vi "Image Processing.vi"() -> ()   [LabVIEW 2016]
uses:
  <vilib>/rvi/Emulation/niFpgaGetClockAttributes.vi
  <vilib>/rvi/Emulation/niFpgaSctlEmulationGetInTimedLoop.vi
  <vilib>/rvi/Emulation/niFpgaEmulationReportErrorSimple.vi
  <vilib>/rvi/Emulation/niFpgaProcessEmulError.vi
  <vilib>/rvi/eio/common/nirviEmuTemplateMethod_errors.vi
  <vilib>/rvi/interface/RandomDataEmulation/niFpgaRandomDataHandleErrors.vi
  <vilib>/rvi/DataTransferAndStorage/Container/Common/niFpgaContainerGetUniqueNameForEmu.vi
  <vilib>/rvi/DataTransferAndStorage/Container/Common/niFpgaContainerSetEmuInfo.vi
  <vilib>/rvi/eio/common/nirviEmuReportErrorAndStop.vi
  <vilib>/rvi/DataTransferAndStorage/Container/Common/niFpgaContainerExecOnDevCompGetState.vi
  <vilib>/rvi/Emulation/niFpgaEmulationIsFPGAContextNoSignature.vi
  <vilib>/rvi/errors/niFpgaSetErrorForExecOnDevCompSimple.vi
  <vilib>/rvi/FIFO/Fifo_Resource/nirvififoEmulationSetSize.vi
  <vilib>/rvi/FIFO/Fifo_Resource/nirviFifoEmulationQueueMgr.vi
  <instcachedir>/0/nirviFifoEmulationQueueMgr_E5CAEC123FF24DC58D834DCA3CDAA9B5.lvgen/nirviFifoEmulationQueueMgr_E5CAEC123FF24DC58D834DCA3CDAA9B5_002.vi
  <vilib>/rvi/FIFO/Fifo_Resource/nirvififoEmulationDetermineInputValidOut.vi
  <vilib>/rvi/FIFO/Fifo_Resource/nirvififoEmulationCreateLock.vi
  <vilib>/rvi/FIFO/Fifo_Resource/nirvififoEmulationObtainLock.vi
  <vilib>/rvi/FIFO/Fifo_Resource/nirvififoEmulationReleaseLock.vi
  <vilib>/rvi/occurrence/nirviWaitOnOccurrenceBase.vi
  <vilib>/rvi/errors/nirviReportUnexpectedCaseInternalError.vi
  <vilib>/rvi/errors/nirviReportUnexpectedCaseInternalError (U32).vi
  <vilib>/Utility/error.llb/Clear Errors.vi
  <vilib>/rvi/Emulation/niFpgaCriticalErrorInLSC.vi
  <vilib>/eio/EIONode/EIONode.xnode
  <vilib>/rvi/DataTransferAndStorage/Container/XNode/niFpgaContainer.xnode
  <vilib>/rvi/interface/RandomDataEmulation/nirviRandomDataFpgaReadWriteTemplate.vi
  <vilib>/rvi/LocalResourceManager/LocalResourceManager.xnode
  <vilib>/rvi/FIFO/Fifo_Resource/niFpgaFifoEmulationRefIn.vi
panel:
  out "dec deHeight":u16
  out "dec deWidth":u16
  out "dec Height":u16
  out "dec Width":u16
  out "Width":u16=320
  out "Height":u16=240
  out "deHeight":u16=240
  out "deWidth":u16=320
  out "Count":u32
  out "OutputType":u8
  out "CanSendImage":bool=TRUE
  out "Mode LED Status":bool=TRUE
  out "Radio LED Status":bool=TRUE
  out "outputExtreme2":bool=TRUE
  out "outputExtreme1":bool=TRUE
  out "outputDOG2":bool=TRUE
  out "outputDOG1":bool=TRUE
  out "Ready For Output":bool=TRUE
  out "StartOfImage":bool=TRUE
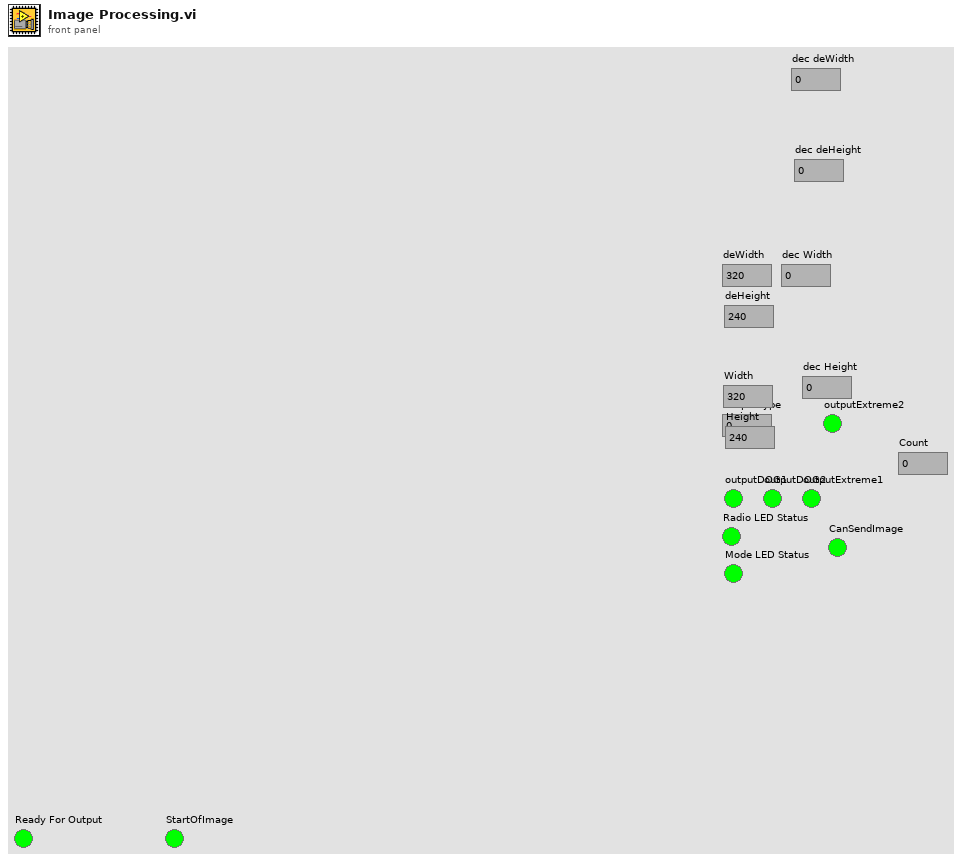
[diagram p1: front panel]
types:
  T1 = cluster{"curCol":u16, "curRow":u16, "Width":u16, "Height":u16, "Data Out":u8, bool}
  T2 = cluster{"curCol":u16, "curRow":u16, "Width":u16, "Height":u16, "GaussianFilterData out":u8, "DV out":bool}
  T3 = cluster{"t":i16, "t":i16, "deWidth":u16, "deHeight":u16, "GaussianFilterData out":u8, "DV out":bool}
  T4 = cluster{"t":i16, "t":i16, "deWidth":u16, "deHeight":u16, "Data Out":u8, "DV out":bool}
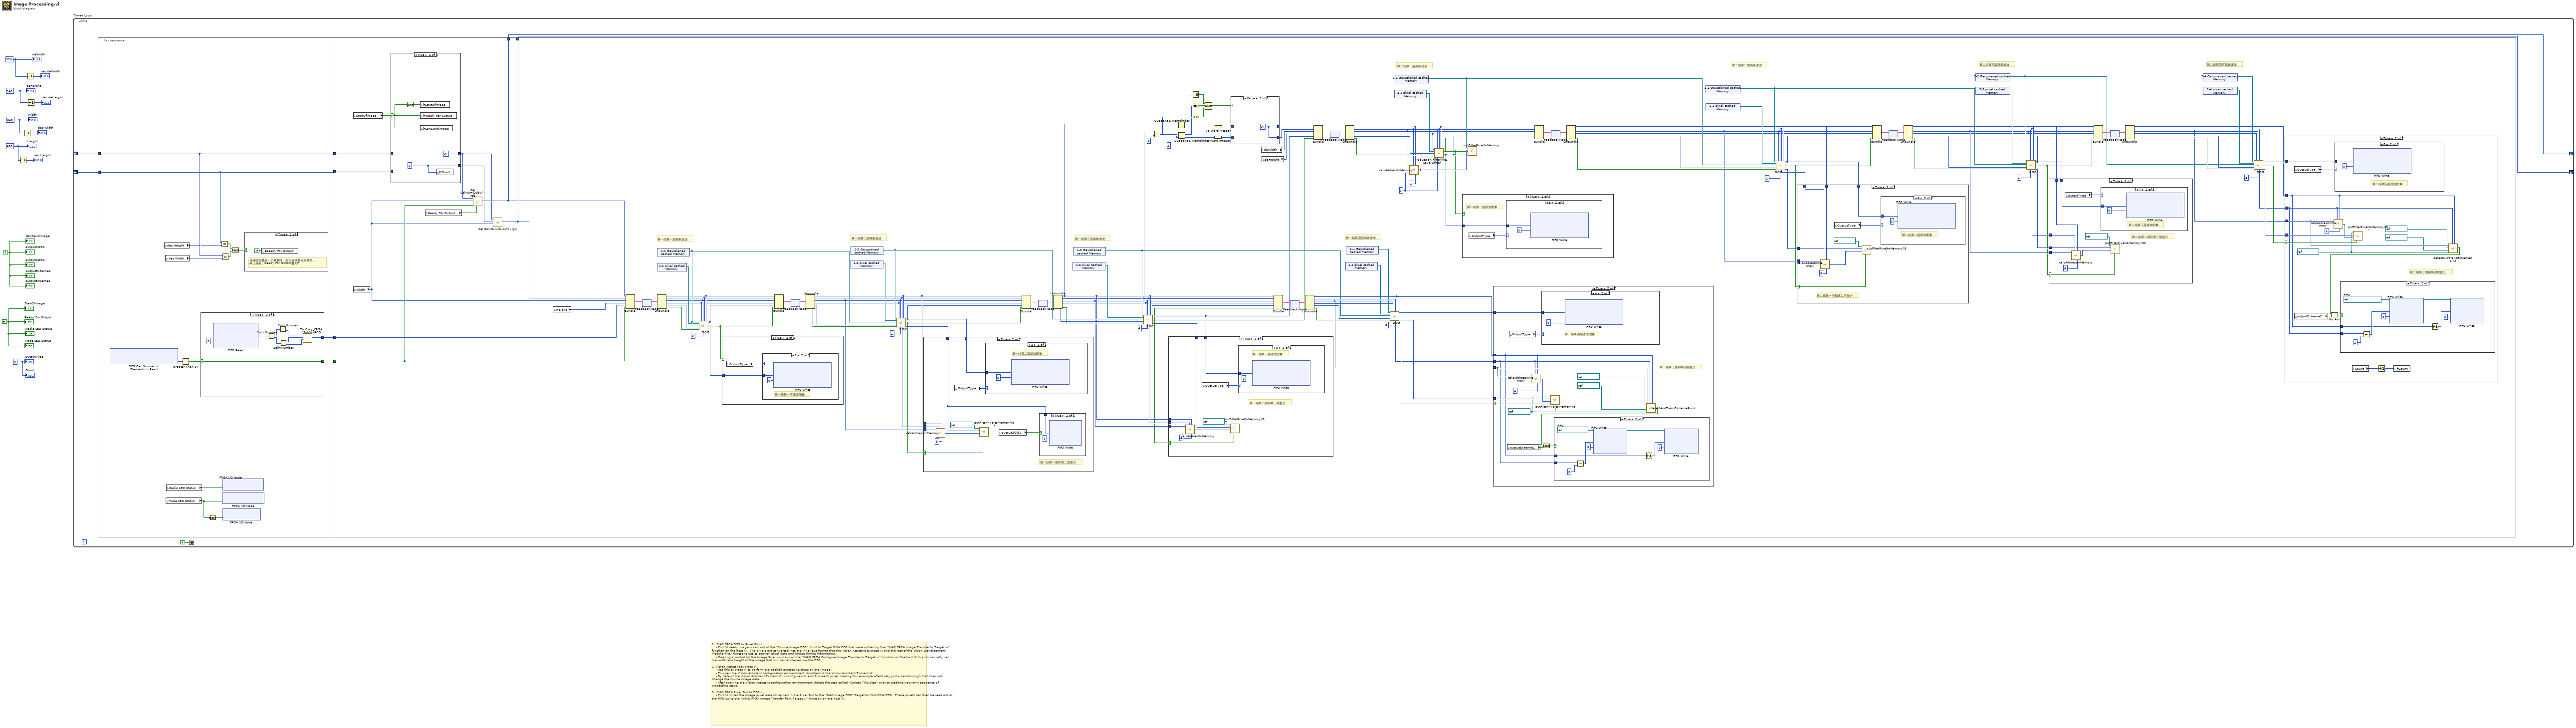
[diagram p0: block diagram]
diagram:
  w5 = i16 480
  w8 = i16 640
  w1 = i16 240
  w3 = i16 320
  w9 = FALSE
  w10 = i16 0
  w11 = TRUE ("Ready For Output")
  # "1. IMAQ FPGA FIFO to Pixel Bus.vi\n    - This VI reads image pixels out of the \"Source Image FIFO\"  Host to Target DMA FIFO that were written by the \"IMAQ FPGA Image Transfer to Target.vi\" function on the host VI.  The pixels are converted into the Pixel Bus format that the Vision Assistant Express VI and the rest of the Vision Development Module FPGA functions use to convey pixel data and image timing information.\n    - Creating a control for the Image Size input allows the \"IMAQ FPGA Configure Image Transfer to Target.vi\" function on the host VI to automatically set the width and height of the image that will be transferred via the FIFO.\n\n2. Vision Assistant Express VI\n    - Use this Express VI to perform the desired processing steps on the image.\n    - To open the Vision Assistant configuration environment, double-click the Vision Assistant Express VI.\n    - By default the Vision Assistant Express VI is configured to add 0 to each pixel, making this example effectively just a pass-through that does not change the source image data.\n    - After opening the Vision Assistant configuration environment, delete the step called \"Delete This Step\" prior to creating your own sequence of processing steps.\n\n3. IMAQ FPGA Pixel Bus to FIFO.vi\n    - This VI writes the image pixel data contained in the Pixel Bus to the \"Dest Image FIFO\" Target to Host DMA FIFO.  These pixels can then be read out of the FIFO using the \"IMAQ FPGA Image Transfer from Target.vi\" function on the host VI."
  n1 = Decrement(x=w5) -> (x-1=→"dec Height":i16)
  n2 = Decrement(x=w8) -> (x-1=→"dec Width":i16)
  n3 = Decrement(x=w3) -> (x-1=→"dec deWidth":i16)
  n4 = Decrement(x=w1) -> (x-1=→"dec deHeight":i16)
  n5 = while "Timed Loop" {
    shift-right: [w12] -> _
    shift-left: _ -> [w14]
    shift-right: [w13] -> _
    shift-left: _ -> [w16]
    stop <- FALSE stop-if-true
    n6 = flat-sequence {
      tunnel: [w29] -> w19
      tunnel: [w28] -> w18
      tunnel: [w23] -> w17
      tunnel: w16 -> [w23]
      tunnel: [w24] -> w15
      tunnel: w14 -> [w24]
      tunnel: w19 -> [w115]
      tunnel: w18 -> [w114]
      tunnel: w17 -> [w49]
      tunnel: w15 -> [w48]
      tunnel: [w55] -> w12
      tunnel: [w54] -> w13
      frame #0 {
        n7 = xnode ("FIFO Get Number of Elements to Read")() -> ("Number of Elements to Read"=w31:u32)  [unwired: 1 in, 1 out]
        n8 = local read "dec Height"() -> (w22:u16)
        n9 = local read "dec Width"() -> (w21:u16)
        n10 = local read "Mode LED Status"() -> (w34:bool)
        n11 = local read "Radio LED Status"() -> (w32:bool)
        n12 = Greater Than 0?(x=w31) -> (x > 0?=w30:bool)
        n13 = case shown="True" w30 {
          selector: w30 -> [w36 w37]
          tunnel: [_ w38] -> w29
          tunnel: [w36 w37] -> w28
          frame False {
          }
          frame True {
            n14 = xnode ("FIFO Read")("Timeout"=0) -> ("Element"=w45:u32)  [unwired: 1 in, 2 out]
            n15 = Split Number(x=w45) -> (hi(x)=w43:u16, lo(x)=w44:u16)
            n16 = Split Number(x=w43) -> (lo(x)=w42:u8)  [unwired: 1 out]
            n17 = Split Number(x=w44) -> (hi(x)=w41:u8, lo(x)=w40:u8)
            n18 = call "To Gray_FPGA (SubVI)-RGB.vi"("B"=w40, "G"=w41, "R"=w42) -> ("Data Out"=w38:u8)  [unwired: 8 in]
          }
        }
        n19 = Not(x=w34) -> (.not. x?=w33:bool)
        n20 = Equal?(x=w24, y=w22) -> (x = y?=w25:bool)
        n21 = Equal?(x=w23, y=w21) -> (x = y?=w26:bool)
        n22 = xnode "FPGA I/O Node"("Radio LED Green"=w32) -> ()  [unwired: 1 in, 1 out]
        n23 = xnode "FPGA I/O Node"("Mode LED Green"=w34) -> ()  [unwired: 1 in, 1 out]
        n24 = xnode "FPGA I/O Node"("Mode LED Red"=w33) -> ()  [unwired: 1 in, 1 out]
        n25 = And(x=w25, y=w26) -> (x .and. y?=w27:bool)
        n26 = case shown="True" w27 {
          frame False {
          }
          frame True {
            # "当接收完最后一个像素时，由于后续差分未做完，\n停止接收，Ready For Output置为F"
            n27 = local write "Ready For Output"(FALSE ("Ready For Output")) -> ()
          }
        }
      }
      frame #1 {
        w138 = u32 2 ("y")
        w146 = u8 0 ("delayRowCount")
        # "第一组第一层高斯滤波"
        # "第一组第二层高斯滤波"
        # "第一组第三层高斯滤波"
        # "第二组第一层高斯滤波"
        # "第一组第四层高斯滤波"
        # "第二组第二层高斯滤波"
        # "第二组第三层高斯滤波"
        # "第二组第四层高斯滤波"
        n28 = local read "StartOfImage"() -> (w50:bool)
        n29 = local read "Width"() -> (w47:u16)
        n30 = case shown="True" w50 {
          selector: w50 -> [_ w196]
          tunnel: w49 -> [w194 _]
          tunnel: w48 -> [w193 _]
          tunnel: [w194 i16 -1] -> w52
          tunnel: [w193 w195] -> w51
          frame False {
          }
          frame True {
            w195 = i16 0
            n31 = Not(x=w196) -> (.not. x?=w197:bool)
            n32 = local write "StartOfImage"(w197) -> ()
            n33 = local write "Ready For Output"(w196) -> ()
            n34 = local write "CanSendImage"(w196) -> ()
            n35 = local write "Count"(w195) -> ()
          }
        }
        n36 = local read "Ready For Output"() -> (w53:bool)
        n37 = call "Cal ColNum(SubVI) - rgb.vi"("Ready For Input"=w53, "DV"=w114, "Width"=w47, "preCol"=w52) -> ("curCol"=w54:u16)  [unwired: 7 in]
        n38 = call "Cal RowNum(SubVI) - rgb.vi"("Width"=w47, "preRow"=w51, "preCol"=w52) -> ("curRow"=w55:u16)  [unwired: 8 in]
        n39 = local read "Height"() -> (w46:u16)
        n40 = Bundle("curCol"=w54, "curRow"=w55, "Width"=w47, "Height"=w46, "Data Out"=w115, w114) -> (w119:T1)  [unwired: 1 in]
        n41 = feedback #1() -> (w118:T1)  [unwired: 1 in]
        n42 = feedback-in #1(w119) -> ()
        n43 = xnode "1-1 Gaussianed cached Memory"() -> ("Memory Out"=w126:refnum<k21>)
        n44 = xnode "1-1 pixel cached Memory"() -> ("Memory Out"=w121:refnum<k21>)
        n45 = Unbundle(w118) -> ("curCol"=w111:u16, "curRow"=w110:u16, "Width"=w109:u16, "Height"=w108:u16, "Data Out"=w117:u8, w116:bool)
        n46 = call "DOG.vi"("Gaussianed cached Memory"=w126, "pixel cached Memory"=w121, "preGaussianed cached Memory"=w126, "Data in"=w117, "DV in"=w116, "Height"=w108, "Width"=w109, "DelayRowCount"=i16 0, "Rows"=w110, "Cols"=w111) -> ("GaussianFilterData out"=w107:u8, "DV out"=w106:bool)  [unwired: 6 in, 2 out]
        n47 = case shown="True" w106 {
          tunnel: w107 -> [_ w200]
          frame False {
          }
          frame True {
            n48 = local read "OutputType"() -> (w199:u8)
            n49 = case shown="1" w199 {
              tunnel: w200 -> [_ w201]
              frame 0, Default {
              }
              frame 1 {
                # "第一组第一层滤波图像"
                n50 = xnode ("FIFO Write")("Element"=w201, "Timeout"=0) -> ()  [unwired: 1 in, 2 out]
              }
            }
          }
        }
        n51 = Bundle("curCol"=w111, "curRow"=w110, "Width"=w109, "Height"=w108, "GaussianFilterData out"=w107, "DV out"=w106) -> (w112:T2)  [unwired: 1 in]
        n52 = feedback #2() -> (w113:T2)  [unwired: 1 in]
        n53 = feedback-in #2(w112) -> ()
        n54 = Unbundle(w113) -> ("curCol"=w103:u16, "curRow"=w102:u16, "Width"=w101:u16, "Height"=w100:u16, "GaussianFilterData out"=w125:u8, "DV out"=w124:bool)
        n55 = xnode "1-2 Gaussianed cached Memory"() -> ("Memory Out"=w141:refnum<k21>)
        n56 = xnode "1-2 pixel cached Memory"() -> ("Memory Out"=w127:refnum<k21>)
        n57 = call "DOG.vi"("Gaussianed cached Memory"=w141, "pixel cached Memory"=w127, "preGaussianed cached Memory"=w126, "Data in"=w125, "DV in"=w124, "Height"=w100, "Width"=w101, "DelayRowCount"=i16 2, "Rows"=w102, "Cols"=w103) -> ("out Row"=w122:u16, "GaussianFilterData out"=w99:u8, "DV out"=w98:bool, "DOG Out"=w123:i8)  [unwired: 6 in]
        n58 = case shown="True" w98 {
          selector: w98 -> [_ w206]
          tunnel: w99 -> [_ w213]
          tunnel: w123 -> [_ w204]
          tunnel: w101 -> [_ w212]
          tunnel: w122 -> [_ w211]
          tunnel: w103 -> [_ w210]
          frame False {
          }
          frame True {
            # "第一组第一层和第二层差分"
            n59 = call "calcAddressInMemory.vi"("Width"=w212, "Rows"=w211, "Cols"=w210, "divider"=u8 8) -> ("addressInMemory"=w208:u16)  [unwired: 5 in]
            n60 = local read "OutputType"() -> (w205:u8)
            n61 = call "putFilterPixeltoMemory(I8).vi"("DV in"=w206, "addressInMemory"=w208, "Data In"=w204, "Memory in"=refnum<k21> "DOG1-1") -> ()  [unwired: 8 in]
            n62 = case shown="2" w205 {
              tunnel: w213 -> [_ w216]
              frame 0, Default {
              }
              frame 2 {
                # "第一组第二层滤波图像"
                n63 = xnode ("FIFO Write")("Element"=w216, "Timeout"=0) -> ()  [unwired: 1 in, 2 out]
              }
            }
            n64 = local read "outputDOG1"() -> (w203:bool)
            n65 = case shown="True" w203 {
              tunnel: w204 -> [_ w215]
              frame False {
              }
              frame True {
                n66 = xnode ("FIFO Write")("Element"=w215, "Timeout"=0) -> ()  [unwired: 1 in, 2 out]
              }
            }
          }
        }
        n67 = Bundle("curCol"=w103, "curRow"=w102, "Width"=w101, "Height"=w100, "GaussianFilterData out"=w99, "DV out"=w98) -> (w105:T2)  [unwired: 1 in]
        n68 = feedback #3() -> (w104:T2)  [unwired: 1 in]
        n69 = feedback-in #3(w105) -> ()
        n70 = Unbundle(w104) -> ("curCol"=w95:u16, "curRow"=w94:u16, "Width"=w93:u16, "Height"=w92:u16, "GaussianFilterData out"=w143:u8, "DV out"=w144:bool)
        n71 = xnode "1-3 pixel cached Memory"() -> ("Memory Out"=w142:refnum<k21>)
        n72 = xnode "1-3 Gaussianed cached Memory"() -> ("Memory Out"=w158:refnum<k21>)
        n73 = call "DOG.vi"("Gaussianed cached Memory"=w158, "pixel cached Memory"=w142, "preGaussianed cached Memory"=w141, "Data in"=w143, "DV in"=w144, "Height"=w92, "Width"=w93, "DelayRowCount"=i16 4, "Rows"=w94, "Cols"=w95) -> ("out Row"=w129:u16, "GaussianFilterData out"=w81:u8, "DV out"=w80:bool, "DOG Out"=w130:i8)  [unwired: 6 in]
        n74 = Subtract(x=w94, y=i16 6) -> (x-y=w133:u16)
        n75 = case shown="True" w80 {
          selector: w80 -> [_ w222]
          tunnel: w81 -> [_ w230]
          tunnel: w130 -> [_ w223]
          tunnel: w129 -> [_ w226]
          tunnel: w93 -> [_ w225]
          tunnel: w95 -> [_ w224]
          frame False {
          }
          frame True {
            # "第一组第二层和第三层差分"
            n76 = call "calcAddressInMemory.vi"("Width"=w225, "Rows"=w226, "Cols"=w224, "divider"=u8 6) -> ("addressInMemory"=w228:u16)  [unwired: 5 in]
            n77 = local read "OutputType"() -> (w221:u8)
            n78 = call "putFilterPixeltoMemory(I8).vi"("DV in"=w222, "addressInMemory"=w228, "Data In"=w223, "Memory in"=refnum<k21> "DOG1-2") -> ()  [unwired: 8 in]
            n79 = case shown="3" w221 {
              tunnel: w230 -> [_ w231]
              frame 0, Default {
              }
              frame 3 {
                # "第一组第三层滤波图像"
                n80 = xnode ("FIFO Write")("Element"=w231, "Timeout"=0) -> ()  [unwired: 1 in, 2 out]
              }
            }
          }
        }
        n81 = Quotient & Remainder(x=w95, y=w138) -> (x-y*floor(x/y)=w132:u32, floor(x/y)=w88:u32)
        n82 = Quotient & Remainder(x=w133, y=w138) -> (x-y*floor(x/y)=w131:u32, floor(x/y)=w86:u32)
        n83 = Equal To 0?(x=w132) -> (x = 0?=w137:bool)
        n84 = Equal To 0?(x=w131) -> (x = 0?=w136:bool)
        n85 = Greater Or Equal To 0?(x=w133) -> (x >= 0?=w135:bool)
        n86 = Compound Arithmetic op=AND(w137, w136, w135) -> (w134:bool)
        n87 = To Word Integer(number=w86) -> (16bit integer=w87:i16)
        n88 = To Word Integer(number=w88) -> (16bit integer=w89:i16)
        n89 = case shown="False" w134 {
          tunnel: [w218 w220] -> w85
          tunnel: w89 -> [_ w220]
          tunnel: [w218 w219] -> w84
          tunnel: w87 -> [_ w219]
          frame False {
            w218 = i16 -1 ("t")
          }
          frame True {
          }
        }
        n90 = local read "deWidth"() -> (w83:u16)
        n91 = local read "deHeight"() -> (w82:u16)
        n92 = Bundle("curCol"=w95, "curRow"=w94, "Width"=w93, "Height"=w92, "GaussianFilterData out"=w81, "DV out"=w80) -> (w96:T2)  [unwired: 1 in]
        n93 = feedback #4() -> (w97:T2)  [unwired: 1 in]
        n94 = feedback-in #4(w96) -> ()
        n95 = Unbundle(w97) -> ("curCol"=w148:u16, "curRow"=w162:u16, "Width"=w150:u16, "Height"=w161:u16, "GaussianFilterData out"=w164:u8, "DV out"=w163:bool)
        n96 = Bundle("t"=w85, "t"=w84, "deWidth"=w83, "deHeight"=w82, "GaussianFilterData out"=w81, "DV out"=w80) -> (w90:T3)  [unwired: 1 in]
        n97 = feedback #5() -> (w91:T3)  [unwired: 1 in]
        n98 = feedback-in #5(w90) -> ()
        n99 = Unbundle(w91) -> ("t"=w77:i16, "t"=w76:i16, "deWidth"=w75:u16, "deHeight"=w74:u16, "GaussianFilterData out"=w154:u8, "DV out"=w155:bool)
        n100 = xnode "1-4 pixel cached Memory"() -> ("Memory Out"=w159:refnum<k21>)
        n101 = xnode "1-4 Gaussianed cached Memory"() -> ("Memory Out"=w160:refnum<k21>)
        n102 = call "DOG.vi"("Gaussianed cached Memory"=w160, "pixel cached Memory"=w159, "preGaussianed cached Memory"=w158, "Data in"=w164, "DV in"=w163, "Height"=w161, "Width"=w150, "DelayRowCount"=i16 6, "Rows"=w162, "Cols"=w148) -> ("out Row"=w149:u16, "GaussianFilterData out"=w156:u8, "DV out"=w152:bool, "DOG Out"=w151:i8)  [unwired: 6 in]
        n103 = xnode "2-1 Gaussianed cached Memory"() -> ("Memory Out"=w169:refnum<k21>)
        n104 = xnode "2-1 pixel cached Memory"() -> ("Memory Out"=w153:refnum<k21>)
        n105 = call "calcAddressInMemory.vi"("Width"=w75, "Rows"=w76, "delayRowCount"=w146, "Cols"=w77, "divider"=u8 4) -> ("addressInMemory"=w147:u16)  [unwired: 4 in]
        n106 = call "Gaussian Filter(Pic1 LevelOther).vi"("Height"=w74, "Width"=w75, "Rows"=w76, "Cols"=w77, "Memory in"=w153, "Data in"=w154, "DV in"=w155, "Address In"=w147, "DelayRowCount"=w146) -> ("DV out"=w72:bool, "Data Out"=w73:u8)  [unwired: 4 in, 1 out]
        n107 = case shown="True" w72 {
          tunnel: w73 -> [_ w234]
          frame False {
          }
          frame True {
            # "第二组第一层滤波图像"
            n108 = local read "OutputType"() -> (w233:u8)
            n109 = case shown="5" w233 {
              tunnel: w234 -> [_ w235]
              frame 0, Default {
              }
              frame 5 {
                n110 = xnode ("FIFO Write")("Element"=w235, "Timeout"=0) -> ()  [unwired: 1 in, 2 out]
              }
            }
          }
        }
        n111 = call "putFilterPixeltoMemory.vi"("Data In"=w73, "DV in"=w72, "addressInMemory"=w147, "Memory in"=w169) -> ()
        n112 = case shown="True" w152 {
          selector: w152 -> [_ w247]
          tunnel: w156 -> [_ w251]
          tunnel: w151 -> [_ w248]
          tunnel: w150 -> [_ w246]
          tunnel: w149 -> [_ w240]
          tunnel: w148 -> [_ w241]
          frame False {
          }
          frame True {
            w243 = refnum<k21> "DOG1-3" ("Memory in")
            # "第一组第三层和第四层差分"
            n113 = local read "outputExtreme1"() -> (w238:bool)
            n114 = local read "OutputType"() -> (w242:u8)
            n115 = call "calcAddressInMemory.vi"("Width"=w246, "Rows"=w240, "Cols"=w241, "divider"=u8 4) -> ("addressInMemory"=w249:u16)  [unwired: 5 in]
            n116 = case shown="4" w242 {
              tunnel: w251 -> [_ w262]
              frame 0, Default {
              }
              frame 4 {
                # "第一组第四层滤波图像"
                n117 = xnode ("FIFO Write")("Element"=w262, "Timeout"=0) -> ()  [unwired: 1 in, 2 out]
              }
            }
            n118 = call "putFilterPixeltoMemory(I8).vi"("DV in"=w247, "addressInMemory"=w249, "Data In"=w248, "Memory in"=w243) -> ()  [unwired: 8 in]
            n119 = call "detectAndTransExtremePoint.vi"("Col"=w241, "Row"=w240, "Level3 Memory"=w243, "Level2 Memory"=refnum<k21> "DOG1-2" ("Memory In"), "Level1 Memory"=refnum<k21> "DOG1-1" ("Memory In"), "Width"=w246) -> ("isExtreme?"=w237:bool)  [unwired: 5 in]
            n120 = And(x=w237, y=w238) -> (x .and. y?=w239:bool)
            n121 = case shown="True" w239 {
              tunnel: w240 -> [_ w259]
              tunnel: w241 -> [_ w253]
              frame False {
              }
              frame True {
                w252 = refnum<k21> "extreme FIFO"  # FIFO
                n122 = Subtract(x=w259, y=u16 2) -> (x-y=w257:u16)
                n123 = xnode ("FIFO Write")("Element"=w257, "Timeout"=0, "FIFO In"=w252) -> ("FIFO Out"=w255:refnum<k21>)  [unwired: 1 out]
                n124 = Increment(x=w253) -> (x+1=w254:u16)
                n125 = xnode ("FIFO Write")("Element"=w254, "Timeout"=0, "FIFO In"=w255) -> ()  [unwired: 2 out]
              }
            }
          }
        }
        n126 = Bundle("t"=w77, "t"=w76, "deWidth"=w75, "deHeight"=w74, "Data Out"=w73, "DV out"=w72) -> (w79:T4)  [unwired: 1 in]
        n127 = feedback #6() -> (w78:T4)  [unwired: 1 in]
        n128 = feedback-in #6(w79) -> ()
        n129 = Unbundle(w78) -> ("t"=w69:i16, "t"=w68:i16, "deWidth"=w67:u16, "deHeight"=w66:u16, "Data Out"=w168:u8, "DV out"=w167:bool)
        n130 = xnode "2-2 Gaussianed cached Memory"() -> ("Memory Out"=w176:refnum<k21>)
        n131 = xnode "2-2 pixel cached Memory"() -> ("Memory Out"=w170:refnum<k21>)
        n132 = call "DOG.vi"("Gaussianed cached Memory"=w176, "pixel cached Memory"=w170, "preGaussianed cached Memory"=w169, "Data in"=w168, "DV in"=w167, "Height"=w66, "Width"=w67, "DelayRowCount"=i16 2, "Rows"=w68, "Cols"=w69) -> ("out Row"=w165:u16, "GaussianFilterData out"=w65:u8, "DV out"=w64:bool, "DOG Out"=w166:i8)  [unwired: 6 in]
        n133 = case shown="True" w64 {
          selector: w64 -> [_ w264]
          tunnel: w166 -> [_ w265]
          tunnel: w65 -> [_ w272]
          tunnel: w69 -> [_ w268]
          tunnel: w165 -> [_ w267]
          tunnel: w67 -> [_ w266]
          frame False {
          }
          frame True {
            # "第二组第一层和第二层差分"
            n134 = call "calcAddressInMemory.vi"("Width"=w266, "Rows"=w267, "Cols"=w268, "divider"=u8 8) -> ("addressInMemory"=w270:u16)  [unwired: 5 in]
            n135 = local read "OutputType"() -> (w263:u8)
            n136 = call "putFilterPixeltoMemory(I8).vi"("DV in"=w264, "addressInMemory"=w270, "Data In"=w265, "Memory in"=refnum<k21> "DOG2-1") -> ()  [unwired: 8 in]
            n137 = case shown="6" w263 {
              tunnel: w272 -> [_ w273]
              frame 0, Default {
              }
              frame 6 {
                # "第二组第二层滤波图像"
                n138 = xnode ("FIFO Write")("Element"=w273, "Timeout"=0) -> ()  [unwired: 1 in, 2 out]
              }
            }
          }
        }
        n139 = Bundle("t"=w69, "t"=w68, "deWidth"=w67, "deHeight"=w66, "GaussianFilterData out"=w65, "DV out"=w64) -> (w70:T3)  [unwired: 1 in]
        n140 = feedback #7() -> (w71:T3)  [unwired: 1 in]
        n141 = feedback-in #7(w70) -> ()
        n142 = Unbundle(w71) -> ("t"=w61:i16, "t"=w60:i16, "deWidth"=w59:u16, "deHeight"=w58:u16, "GaussianFilterData out"=w175:u8, "DV out"=w174:bool)
        n143 = xnode "2-3 Gaussianed cached Memory"() -> ("Memory Out"=w187:refnum<k21>)
        n144 = xnode "2-3 pixel cached Memory"() -> ("Memory Out"=w177:refnum<k21>)
        n145 = call "DOG.vi"("Gaussianed cached Memory"=w187, "pixel cached Memory"=w177, "preGaussianed cached Memory"=w176, "Data in"=w175, "DV in"=w174, "Height"=w58, "Width"=w59, "DelayRowCount"=i16 4, "Rows"=w60, "Cols"=w61) -> ("out Row"=w172:u16, "GaussianFilterData out"=w57:u8, "DV out"=w56:bool, "DOG Out"=w173:i8)  [unwired: 6 in]
        n146 = case shown="True" w56 {
          selector: w56 -> [_ w276]
          tunnel: w57 -> [_ w284]
          tunnel: w173 -> [_ w277]
          tunnel: w59 -> [_ w280]
          tunnel: w172 -> [_ w279]
          tunnel: w61 -> [_ w278]
          frame False {
          }
          frame True {
            # "第二组第二层和第三层差分"
            n147 = local read "OutputType"() -> (w275:u8)
            n148 = call "calcAddressInMemory.vi"("Width"=w280, "Rows"=w279, "Cols"=w278, "divider"=u8 6) -> ("addressInMemory"=w282:u16)  [unwired: 5 in]
            n149 = case shown="7" w275 {
              tunnel: w284 -> [_ w286]
              frame 0, Default {
              }
              frame 7 {
                # "第二组第三层滤波图像"
                n150 = xnode ("FIFO Write")("Element"=w286, "Timeout"=0) -> ()  [unwired: 1 in, 2 out]
              }
            }
            n151 = call "putFilterPixeltoMemory(I8).vi"("DV in"=w276, "addressInMemory"=w282, "Data In"=w277, "Memory in"=refnum<k21> "DOG2-2") -> ()  [unwired: 8 in]
          }
        }
        n152 = Bundle("t"=w61, "t"=w60, "deWidth"=w59, "deHeight"=w58, "GaussianFilterData out"=w57, "DV out"=w56) -> (w62:T3)  [unwired: 1 in]
        n153 = feedback #8() -> (w63:T3)  [unwired: 1 in]
        n154 = feedback-in #8(w62) -> ()
        n155 = Unbundle(w63) -> ("t"=w180:i16, "t"=w179:i16, "deWidth"=w182:u16, "deHeight"=w186:u16, "GaussianFilterData out"=w189:u8, "DV out"=w188:bool)
        n156 = xnode "2-4 Gaussianed cached Memory"() -> ("Memory Out"=w190:refnum<k21>)
        n157 = xnode "2-4 pixel cached Memory"() -> ("Memory Out"=w191:refnum<k21>)
        n158 = call "DOG.vi"("Gaussianed cached Memory"=w190, "pixel cached Memory"=w191, "preGaussianed cached Memory"=w187, "Data in"=w189, "DV in"=w188, "Height"=w186, "Width"=w182, "DelayRowCount"=i16 6, "Rows"=w179, "Cols"=w180) -> ("out Row"=w181:u16, "GaussianFilterData out"=w184:u8, "DV out"=w185:bool, "DOG Out"=w183:i8)  [unwired: 6 in]
        n159 = case shown="True" w185 {
          selector: w185 -> [_ w300]
          tunnel: w184 -> [_ w303]
          tunnel: w183 -> [_ w299]
          tunnel: w182 -> [_ w298]
          tunnel: w181 -> [_ w296]
          tunnel: w180 -> [_ w297]
          frame False {
          }
          frame True {
            w287 = refnum<k21> "DOG2-3" ("Level3 Memory")
            # "第二组第三层和第四层差分"
            n160 = local read "OutputType"() -> (w292:u8)
            n161 = local read "outputExtreme2"() -> (w293:bool)
            n162 = call "calcAddressInMemory.vi"("Width"=w298, "Rows"=w296, "Cols"=w297, "divider"=u8 4) -> ("addressInMemory"=w301:u16)  [unwired: 5 in]
            n163 = case shown="8" w292 {
              tunnel: w303 -> [_ w305]
              frame 0, Default {
              }
              frame 8 {
                # "第二组第四层滤波图像"
                n164 = xnode ("FIFO Write")("Element"=w305, "Timeout"=0) -> ()  [unwired: 1 in, 2 out]
              }
            }
            n165 = local read "Count"() -> (w291:u32)
            n166 = call "putFilterPixeltoMemory(I8).vi"("DV in"=w300, "addressInMemory"=w301, "Data In"=w299, "Memory in"=w287) -> ()  [unwired: 8 in]
            n167 = Increment(x=w291) -> (x+1=w290:u32)
            n168 = local write "Count"(w290) -> ()
            n169 = call "detectAndTransExtremePoint.vi"("Col"=w297, "Row"=w296, "Level3 Memory"=w287, "Level2 Memory"=refnum<k21> "DOG2-2", "Level1 Memory"=refnum<k21> "DOG2-1", "Width"=w298) -> ("isExtreme?"=w294:bool)  [unwired: 5 in]
            n170 = Not And(1:w293, 2:w294) -> (0:w295:bool)
            n171 = case shown="True" w295 {
              tunnel: w296 -> [_ w313]
              tunnel: w297 -> [_ w307]
              frame False {
              }
              frame True {
                w306 = refnum<k21> "extreme FIFO dec"  # FIFO
                n172 = Subtract(x=w313, y=u16 2) -> (x-y=w311:u16)
                n173 = xnode ("FIFO Write")("Element"=w311, "Timeout"=0, "FIFO In"=w306) -> ("FIFO Out"=w309:refnum<k21>)  [unwired: 1 out]
                n174 = Increment(x=w307) -> (x+1=w308:i16)
                n175 = xnode ("FIFO Write")("Element"=w308, "Timeout"=0, "FIFO In"=w309) -> ()  [unwired: 2 out]
              }
            }
          }
        }
      }
    }
  }
  "StartOfImage" <- w11
  "Ready For Output" <- w11
  "outputDOG1" <- w9
  "outputDOG2" <- w9
  "outputExtreme1" <- w9
  "outputExtreme2" <- w9
  "Radio LED Status" <- w11
  "Mode LED Status" <- w11
  "CanSendImage" <- w9
  "OutputType" <- w10
  "Count" <- w10
  "deWidth" <- w3
  "deHeight" <- w1
  "Width" <- w8
  "Height" <- w5
